vi "BenchFromIni.vi"(8 "error in (no error)":errorcluster, 11 "configuration file path":path=path "C:/BytelabsRepository/webapibytegs/RESTServerCfg.ini") -> (0 "error out":errorcluster, 3 "Array":string[](array[string]))   [LabVIEW 2019]
uses:
  <vilib>/Utility/config.llb/Read Key (String).vi
  <vilib>/Utility/config.llb/NI_LVConfig.lvlib
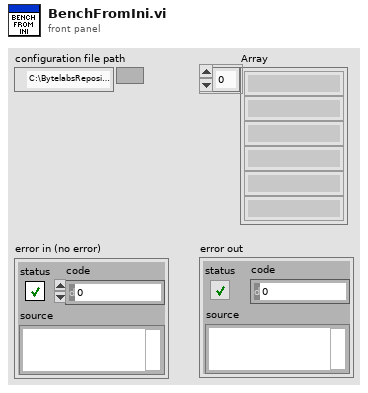
[diagram p1: front panel]
types:
  T1 = typedef "NI_LVConfig.lvlib/Config Data RefNum.ctl" = refnum<k1>
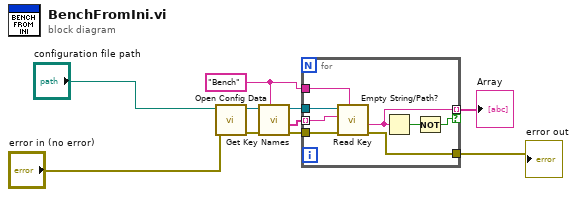
[diagram p0: block diagram]
diagram:
  w5 = "Bench" ("section")
  n1 = call <vilib>:"Open Config Data.vi"("error in (no error)"="error in (no error)", "configuration file path"="configuration file path") -> ("error out"=w6:errorcluster, "refnum"=w2:T1)  [unwired: 7 in, 1 out]
  n2 = call <vilib>:"Get Key Names.vi"("section"=w5, "error in (no error)"=w6, "refnum"=w2) -> ("error out"=w7:errorcluster, "key names"=w8:string[], "refnum out"=w4:T1)  [unwired: 5 in, 1 out]
  n3 = for {
    tunnel: w4 -> [w18]
    tunnel: w7 -> [w17]
    tunnel: [w14] -> w3 mode=indexing if=w12
    tunnel: w5 -> [w16]
    tunnel: w8 -> [w15] mode=indexing
    tunnel: [w11] -> w10
    n4 = call-poly <vilib>:"Read Key.vi"("section"=w16, "error in (no error)"=w17, "key"=w15, "refnum"=w18) -> ("error out"=w11:errorcluster, "value"=w14:string)  [unwired: 4 in, 2 out]
    n5 = Empty String/Path?(string/path=w14) -> (empty?=w13:bool)
    n6 = Not(x=w13) -> (.not. x?=w12:bool)
  }
  "Array" <- w3
  "error out" <- w10
